vi "SC-BG-graphSD.vi"(1 "II channel seq":T1, 2 "I channel seq":T1) -> (0 "Array":cluster{"wavelengths":dbl[], "Tableau":dbl[]}[](array[cluster]))   [LabVIEW 2015]
uses:
  controls/data-cluster.ctl
  globalVarSD.vi
panel:
  out "Graphe XY 2":cluster{dbl[], "wavelengths":dbl[]}(graph)
  out "Graphe XY":cluster{dbl[], "wavelengths":dbl[]}(graph)
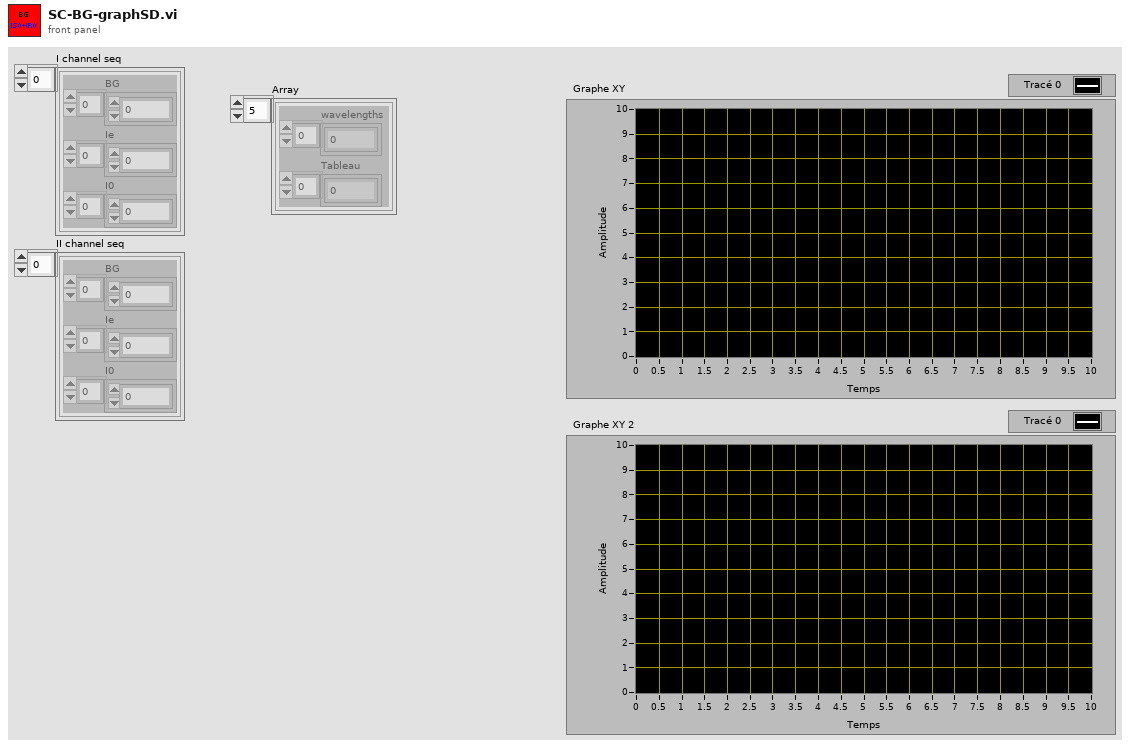
[diagram p1: front panel]
types:
  T1 = typedef "data-cluster.ctl" = cluster{"BG":i32[], "Ie":i32[], "I0":i32[]}[]
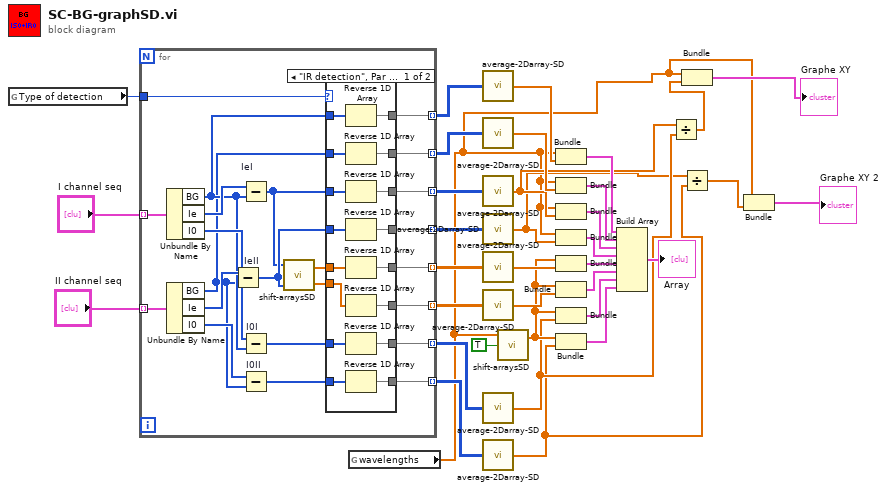
[diagram p0: block diagram]
diagram:
  n1 = global read "globalVarSD.vi" "Type of detection"() -> (w15:enum32{"IR detection", "UV-vis detection"})
  n2 = for {
    tunnel: "I channel seq" -> [w58] mode=indexing
    tunnel: "II channel seq" -> [w57] mode=indexing
    tunnel: [w44] -> w29 mode=indexing
    tunnel: [w46] -> w30 mode=indexing
    tunnel: [w45] -> w31 mode=indexing
    tunnel: [w48] -> w32 mode=indexing
    tunnel: [w52] -> w27 mode=indexing
    tunnel: [w50] -> w26 mode=indexing
    tunnel: w15 -> [w54]
    tunnel: [w38] -> w14 mode=indexing
    tunnel: [w36] -> w12 mode=indexing
    n3 = Unbundle By Name(w58) -> ("BG"=w42:i32[], "Ie"=w56:i32[], "I0"=w43:i32[])
    n4 = Unbundle By Name(w57) -> ("BG"=w40:i32[], "Ie"=w55:i32[], "I0"=w41:i32[])
    n5 = Subtract "IeII"(x=w55, y=w40) -> (x-y=w49:i32[])
    n6 = Subtract "IeI"(x=w56, y=w42) -> (x-y=w47:i32[])
    n7 = Subtract "I0I"(x=w43, y=w42) -> (x-y=w39:i32[])
    n8 = Subtract "I0II"(x=w41, y=w40) -> (x-y=w37:i32[])
    n9 = call "shift-arraysSD.vi"("in2"=w49, "in1"=w47) -> ("out2"=w51:dbl[], "out1"=w53:dbl[])  [unwired: 1 in]
    n10 = case shown="\"IR detection\", Par défaut" w54 {
      tunnel: w53 -> [w67 w79]
      tunnel: [w68 w79] -> w52
      tunnel: w51 -> [w66 w78]
      tunnel: [w65 w78] -> w50
      tunnel: w49 -> [w74 w82]
      tunnel: [w73 w82] -> w48
      tunnel: w47 -> [w72 w81]
      tunnel: [w71 w81] -> w46
      tunnel: w40 -> [w70 w80]
      tunnel: [w69 w80] -> w45
      tunnel: w42 -> [w64 w77]
      tunnel: [w63 w77] -> w44
      tunnel: w39 -> [w62 w76]
      tunnel: [w61 w76] -> w38
      tunnel: w37 -> [w60 w75]
      tunnel: [w59 w75] -> w36
      frame "IR detection", Default {
        n11 = Reverse 1D Array(array=w64) -> (reversed array=w63:i32[])
        n12 = Reverse 1D Array(array=w70) -> (reversed array=w69:i32[])
        n13 = Reverse 1D Array(array=w72) -> (reversed array=w71:i32[])
        n14 = Reverse 1D Array(array=w74) -> (reversed array=w73:i32[])
        n15 = Reverse 1D Array(array=w67) -> (reversed array=w68:dbl[])
        n16 = Reverse 1D Array(array=w66) -> (reversed array=w65:dbl[])
        n17 = Reverse 1D Array(array=w62) -> (reversed array=w61:i32[])
        n18 = Reverse 1D Array(array=w60) -> (reversed array=w59:i32[])
      }
      frame "UV-vis detection" {
      }
    }
  }
  n19 = global read "globalVarSD.vi" "wavelengths"() -> (w2:dbl[])
  n20 = call "average-2Darray-SD.vi"("2D array"=w29) -> ("out array"=w33:dbl[])
  n21 = call "average-2Darray-SD.vi"("2D array"=w31) -> ("out array"=w34:dbl[])
  n22 = call "average-2Darray-SD.vi"("2D array"=w30) -> ("out array"=w9:dbl[])
  n23 = call "average-2Darray-SD.vi"("2D array"=w32) -> ("out array"=w7:dbl[])
  n24 = call "average-2Darray-SD.vi"("2D array"=w27) -> ("out array"=w20:dbl[])
  n25 = call "average-2Darray-SD.vi"("2D array"=w26) -> ("out array"=w19:dbl[])
  n26 = call "average-2Darray-SD.vi"("2D array"=w14) -> ("out array"=w8:dbl[])
  n27 = call "average-2Darray-SD.vi"("2D array"=w12) -> ("out array"=w6:dbl[])
  n28 = call "shift-arraysSD.vi"("inverted"=TRUE, "in1"=w2) -> ("out1"=w11:dbl[])  [unwired: 1 in, 1 out]
  n29 = Bundle("wavelengths"=w2, "out array"=w33) -> (w17:cluster{"wavelengths":dbl[], "out array":dbl[]})  [unwired: 1 in]
  n30 = Bundle("wavelengths"=w2, "out array"=w34) -> (w16:cluster{"wavelengths":dbl[], "out array":dbl[]})  [unwired: 1 in]
  n31 = Bundle("wavelengths"=w2, "out array"=w9) -> (w28:cluster{"wavelengths":dbl[], "out array":dbl[]})  [unwired: 1 in]
  n32 = Bundle("wavelengths"=w2, "out array"=w7) -> (w35:cluster{"wavelengths":dbl[], "out array":dbl[]})  [unwired: 1 in]
  n33 = Bundle("out1"=w11, "out array"=w20) -> (w24:cluster{"out1":dbl[], "out array":dbl[]})  [unwired: 1 in]
  n34 = Bundle("out1"=w11, "out array"=w19) -> (w23:cluster{"out1":dbl[], "out array":dbl[]})  [unwired: 1 in]
  n35 = Bundle("out1"=w11, "out array"=w8) -> (w13:cluster{"out1":dbl[], "out array":dbl[]})  [unwired: 1 in]
  n36 = Bundle("out1"=w11, "out array"=w6) -> (w10:cluster{"out1":dbl[], "out array":dbl[]})  [unwired: 1 in]
  n37 = Build Array(w17, w16, w28, w35, w24, w23, w13, w10) -> (→"Array":cluster{"out1":dbl[], "out array":dbl[]}[])
  n38 = Divide(x=w9, y=w8) -> (x/y=w3:dbl[])
  n39 = Bundle("wavelengths"=w2, w3) -> (→"Graphe XY":cluster{"wavelengths":dbl[], dbl[]})  [unwired: 1 in]
  n40 = Divide(x=w7, y=w6) -> (x/y=w4:dbl[])
  n41 = Bundle("wavelengths"=w2, w4) -> (→"Graphe XY 2":cluster{"wavelengths":dbl[], dbl[]})  [unwired: 1 in]
